vi "Read MLVClient.vi"(8 "error in (no error)":errorcluster, 11 "MongoDB-Client in":refnum<class "MongoDB-Client.lvclass">) -> (0 "error out":errorcluster, 2 "MLVClient":refnum<k24>, 3 "MongoDB-Client out":refnum<class "MongoDB-Client.lvclass">)   [LabVIEW 2016, in "MongoDB-Client.lvlib" / "MongoDB-Client.lvclass"]
uses:
  MongoDB-Client.lvclass
  D:/Users/blume/Desktop/LV/MongoDB-Driver/MLV DLLs/MongoLabVIEW.dll
  LV/MongoDB-Driver/MLV DLLs/MongoLabVIEW.dll
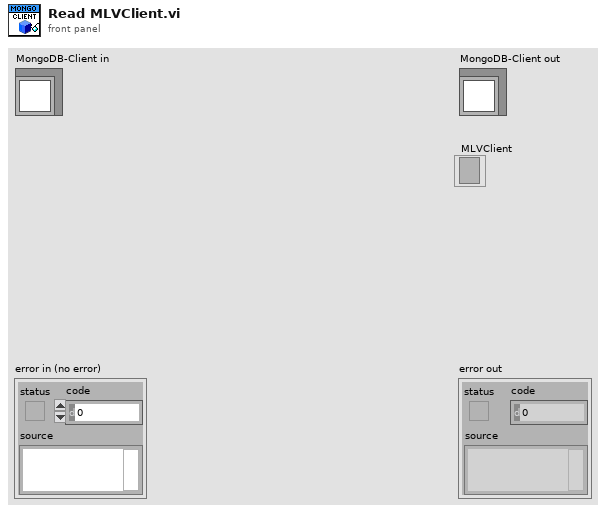
[diagram p1: front panel]
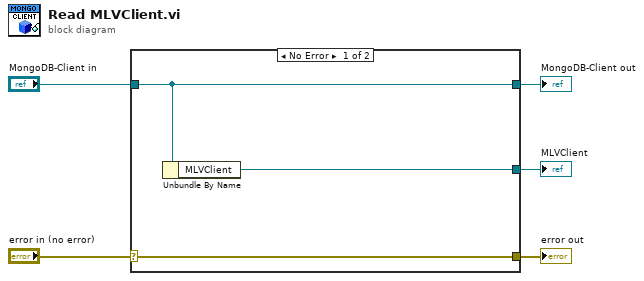
[diagram p0: block diagram]
diagram:
  n1 = case shown="No Error" "error in (no error)" {
    selector: "error in (no error)" -> [w8 w9]
    tunnel: [w8 w9] -> w4
    tunnel: [w7 w10] -> w2
    tunnel: "MongoDB-Client in" -> [w7 w10]
    tunnel: [w6 _] -> w1
    frame No Error {
      n2 = Unbundle By Name(w7) -> ("MLVClient"=w6:refnum<k24>)
    }
    frame Error {
    }
  }
  "error out" <- w4
  "MongoDB-Client out" <- w2
  "MLVClient" <- w1
